vi "ndipolaris Activate All Wired Tools.vi"(8 "error in (no error)":errorcluster, 11 "VISA resource name":refnum<visa-resource-name>) -> (0 "error out":errorcluster, 2 "Port Handles":string[](array[string]), 3 "VISA resource out":refnum<visa-resource-name>)   [LabVIEW 2013]
doc: "This VI will initialize and enable all ports that have an active tool connected to them. An active tool is a wired tool connected either directly to the Polaris or to the Polaris Tool Docking Station."
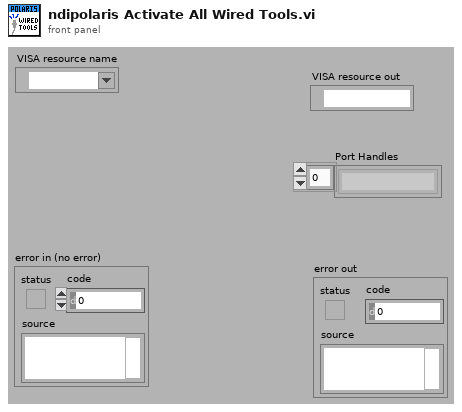
[diagram p1: front panel]
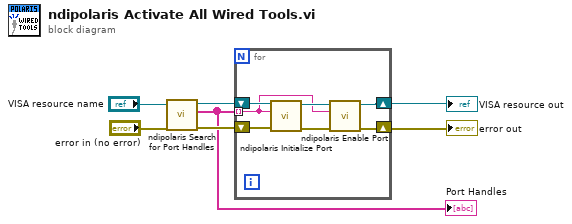
[diagram p0: block diagram]
diagram:
  n1 = call <instrlib>:"ndipolaris Search for Port Handles.vi"("error in (no error)"="error in (no error)", "VISA resource name"="VISA resource name") -> ("error out"=w4:errorcluster, "Handle ID"=w2:string[], "VISA resource out"=w5:refnum<visa-resource-name>)  [unwired: 6 in, 1 out]
  "Port Handles" <- w2
  n2 = for {
    tunnel: w2 -> [w10] mode=indexing
    shift-right: [w9] -> w3
    shift-left: w4 -> [w13]
    shift-right: [w8] -> w1
    shift-left: w5 -> [w14]
    n3 = call <instrlib>:"ndipolaris Initialize Port.vi"("error in (no error)"=w13, "Port Handle"=w10, "VISA resource name"=w14) -> ("error out"=w11:errorcluster, "VISA resource out"=w12:refnum<visa-resource-name>)  [unwired: 7 in]
    n4 = call <instrlib>:"ndipolaris Enable Port.vi"("error in (no error)"=w11, "Port Handle"=w10, "VISA resource name"=w12) -> ("error out"=w9:errorcluster, "VISA resource out"=w8:refnum<visa-resource-name>)  [unwired: 7 in]
  }
  "error out" <- w3
  "VISA resource out" <- w1
